vi "Debug_Convert_Data_to_String.vi"(8 "error in (no error)":errorcluster, 11 "AB_WebService in":refnum<class "AB_WebService.lvclass">) -> (0 "error out":errorcluster, 2 "classData":string, 3 "AB_WebService out":refnum<class "AB_WebService.lvclass">)   [LabVIEW 2020, in "AB_WebService.lvclass"]
uses:
  <vilib>/AppBuilder/AB_Classes/WebService/AB_WebService.lvclass
  <vilib>/AppBuilder/AB_Classes/WebService/AB_WebService.lvclass/AB_WebService.ctl
  <vilib>/AppBuilder/AB_Classes/TargetFile/AB_Targetfile.lvclass
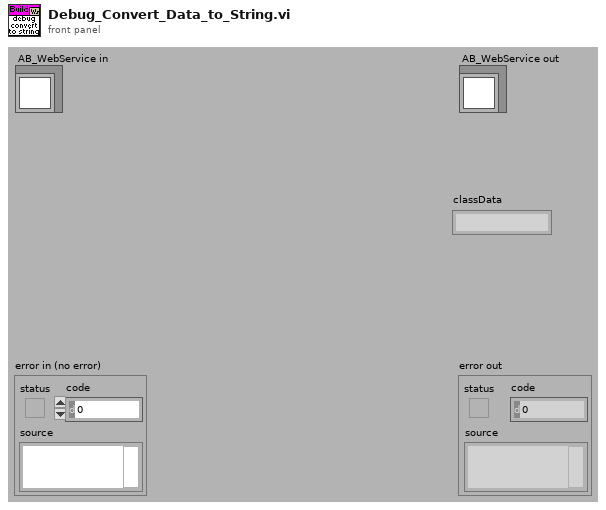
[diagram p1: front panel]
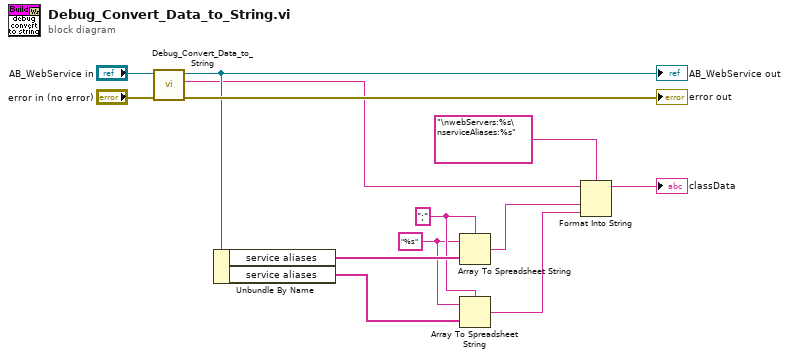
[diagram p0: block diagram]
diagram:
  w4 = ";" ("delimiter (Tab)")
  w3 = "%s" ("format string")
  n1 = call-parent "Debug_Convert_Data_to_String.vi"("error in (no error)"="error in (no error)", "AB_Targetfile in"="AB_WebService in") -> ("error out"=→"error out":errorcluster, "classData"=w8:string, "AB_Targetfile out"=w9:refnum<class "AB_WebService.lvclass">)  [unwired: 7 in]
  "AB_WebService out" <- w9
  n2 = Unbundle By Name(w9) -> ("service aliases"=w6:string[], "service aliases"=w2:string[])
  n3 = Array To Spreadsheet String(delimiter (Tab)=w4, array=w6, 3:w3) -> (spreadsheet string=w5:string)
  n4 = Array To Spreadsheet String(delimiter (Tab)=w4, array=w2, 3:w3) -> (spreadsheet string=w1:string)
  n5 = Format Into String(format string="\nwebServers:%s\nserviceAliases:%s", initial string=w8, w5, w1) -> (resulting string=→"classData":string)  [unwired: 1 in, 1 out]
